vi "20- Arduino based DAQ.vi"() -> ()   [LabVIEW 2019]
uses:
  <vilib>/MakerHub/LINX/Public/Peripherals/Digital/Digital Write 1 Chan.vi
  <vilib>/MakerHub/LINX/Public/Peripherals/Analog/Analog Read 1 Chan.vi
  <vilib>/MakerHub/LINX/Public/Peripherals/Digital/Digital Write N Chans.vi
  <vilib>/MakerHub/LINX/Public/Peripherals/Analog/Analog Read N Chans.vi
  <vilib>/MakerHub/LINX/Private/Local IO/LinxDigitalWrite.vi
  <vilib>/MakerHub/LINX/Public/Utilities/Check Channel.vi
  <vilib>/MakerHub/LINX/Private/Local IO/LinxAnalogRead.vi
  <vilib>/MakerHub/LINX/Public/Utilities/Open Serial.vi
  <vilib>/MakerHub/LINX/Private/Utilties/Generate Error.vi
  <vilib>/MakerHub/LINX/LMH-LINX.lvlib
panel:
  in  "?":bool
  out "Waveform Graph":i32[](graph)
  in  "Plot data from stored value":bool
  in  "Data saving file":path
  in  "Baud Rate Override":u32
  in  "Serial Port":refnum<visa-resource-name>="N/A"
  out "Real time chart":dynamicdata(graph)
  in  "CH4":bool
  in  "CH3":bool
  in  "CH2":bool
  in  "CH1":bool
  in  "Alarm4":dbl
  in  "Alarm2":dbl
  in  "Alarm3":dbl
  in  "Alarm1":dbl
  out "Alarm4":bool
  out "Alarm3":bool
  out "Alarm2":bool
  out "Alarm1":bool
  out "CH4 value":dbl
  out "CH3 value":dbl
  out "CH2 value":dbl
  out "CH1 value":dbl
  out "CH4 meter":dbl(knob) scale=0.0..10.0
  out "CH3 meter":dbl(knob) scale=0.0..10.0
  out "CH2 meter":dbl(knob) scale=0.0..10.0
  out "CH1 meter":dbl(knob) scale=0.0..10.0
  in  "DO4":bool
  in  "DO3":bool
  in  "DO2":bool
  in  "DO1":bool
  # "ARDUINO BASED DATA ACQUISITION SYSTEM(DAQ)"
  # "Arduino configuration"
  # "Select channel"
  # "Set alarm value"
  # "Digital output"
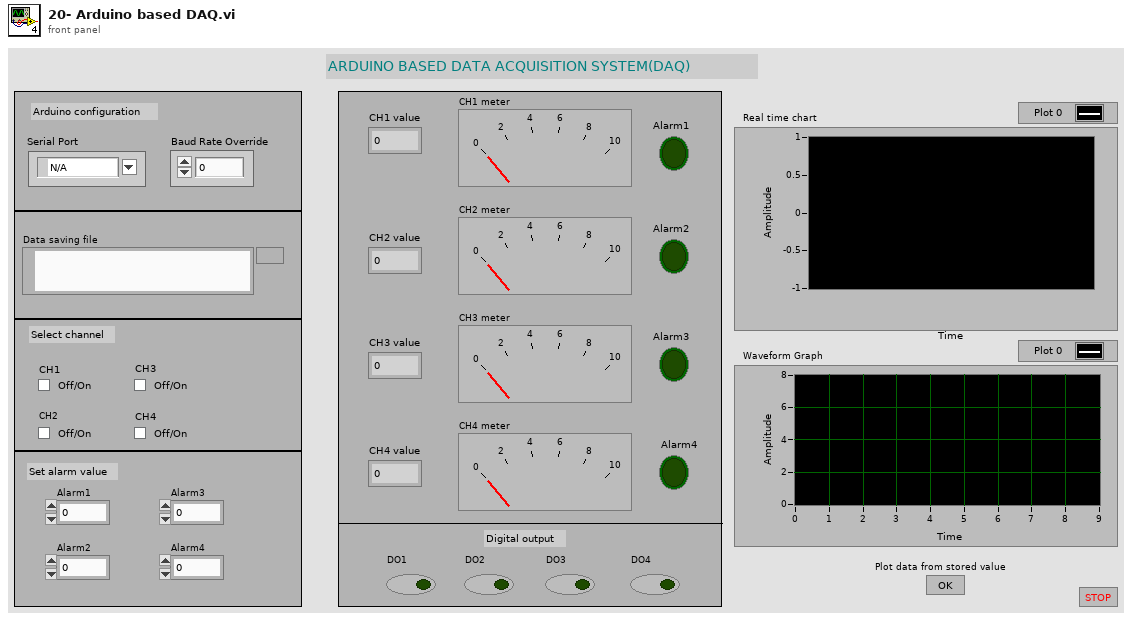
[diagram p1: front panel]
types:
  T1 = enum16{"open", "replace", "create", "open or create", "replace or create", "replace or create with confirmation"}
  T2 = typedef "LMH-LINX.lvlib/LINX Ref.ctl" = cluster{"IO":T3, "Interface":T4, "LINX Device Config":T5}
  T3 = typedef "LMH-LINX.lvlib/Platform.ctl" = enum16{"Remote", "Local"}
  T4 = typedef "LMH-LINX.lvlib/Interface.ctl" = enum16{"Serial", "TCP"}
  T5 = typedef "LMH-LINX.lvlib/Device.lvlib/LINX Device Config.ctl" = cluster{"Interface":T4, "COM Port":refnum<visa-resource-name>, "TCP Configuration":T6, "Device Family":u8, "Device ID":u8, "Device Name":string, "TCP Ref":refnum<k5>, "Channels":T7}
  T6 = typedef "LMH-LINX.lvlib/Device.lvlib/TCP Config.ctl" = cluster{"IP Address":string, "Port":u16}
  T7 = typedef "LMH-LINX.lvlib/Channels.ctl" = cluster{"DI":u8[], "DO":u8[], "AI":u8[], "AO":u8[], "PWM":u8[], "QE":u8[], "UART":u8[], "I2C 2":u8[], "SPI":u8[], "CAN":u8[], "Servo":u8[], "AI Ref (V)":dbl, "AI Resolution (Bits)":u8, "AO Ref (V)":dbl, "AO Resolution (Bits)":u8}
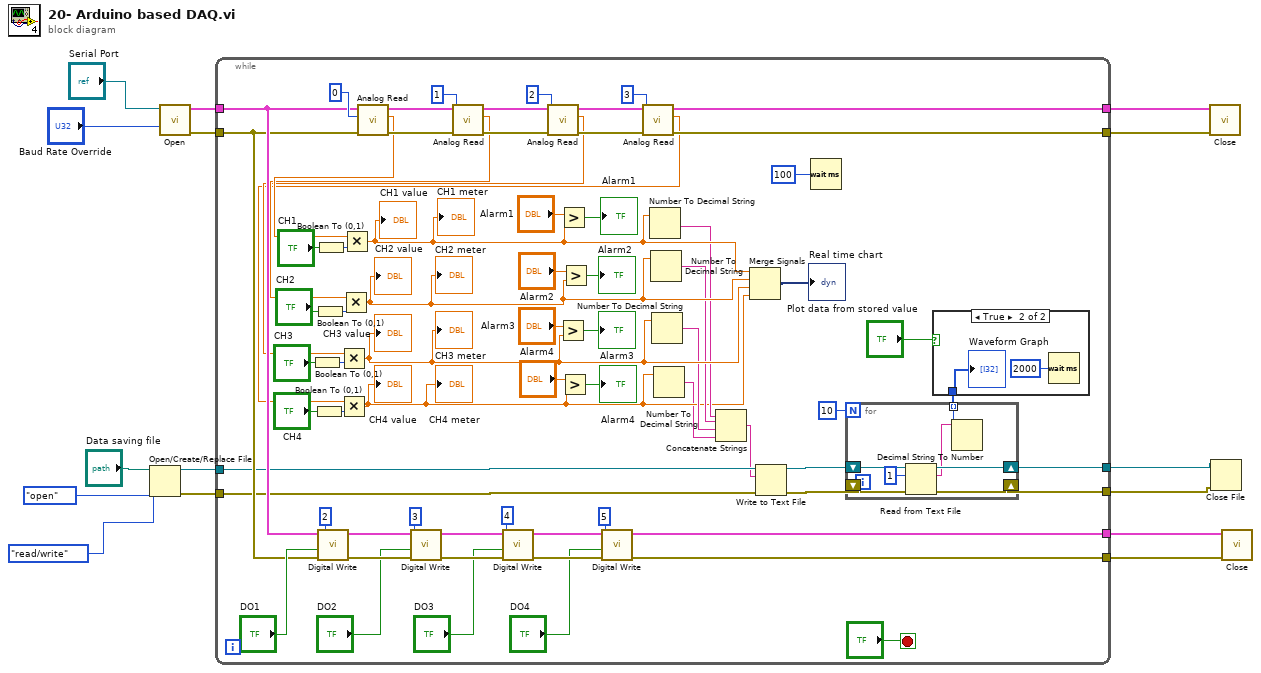
[diagram p0: block diagram]
diagram:
  n1 = Open/Create/Replace File(file path (use dialog)="Data saving file", operation (0:open)=T1."open", access (0:read/write)=enum16{"read/write", "read-only", "write-only"}."read/write") -> (refnum out=w4:refnum<file>, error out=w3:errorcluster)  [unwired: 3 in, 1 out]
  n2 = call-poly <vilib>:"Open.vi"("Baud Rate Override"="Baud Rate Override", "Serial Port"="Serial Port") -> ("Error Out"=w14:errorcluster, "LINX Resource"=w15:T2)  [unwired: 7 in, 1 out]
  n3 = while {
    tunnel: [w62] -> w9
    tunnel: w15 -> [w61]
    tunnel: w14 -> [w59]
    tunnel: [w60] -> w8
    tunnel: [w58] -> w13
    tunnel: [w57] -> w12
    tunnel: w4 -> [w35]
    tunnel: w3 -> [w34]
    tunnel: [w21] -> w2
    tunnel: [w19] -> w1
    stop <- "?" stop-if-true
    n4 = Boolean To (0,1)(Boolean="CH3") -> (0, 1=w42:i16)
    n5 = Boolean To (0,1)(Boolean="CH4") -> (0, 1=w41:i16)
    n6 = Boolean To (0,1)(Boolean="CH2") -> (0, 1=w43:i16)
    n7 = Boolean To (0,1)(Boolean="CH1") -> (0, 1=w44:i16)
    n8 = call-poly <vilib>:"Digital Write.vi"("Error In"=w59, "Output Value"="DO1", "DO Channel"=u8 2, "LINX Resource"=w61) -> ("Error Out"=w77:errorcluster, "LINX Resource"=w80:T2)  [unwired: 6 in]
    n9 = call-poly <vilib>:"Analog Read.vi"("Error In"=w59, "Analog Channel"=u8 0, "LINX Resource"=w61) -> ("Error Out"=w83:errorcluster, "Voltage"=w48:dbl, "LINX Resource"=w86:T2)  [unwired: 5 in, 1 out]
    n10 = Multiply(x=w48, y=w44) -> (x*y=w33:dbl)
    "CH1 meter" <- w33
    "CH1 value" <- w33
    n11 = call-poly <vilib>:"Digital Write.vi"("Error In"=w77, "Output Value"="DO2", "DO Channel"=u8 3, "LINX Resource"=w80) -> ("Error Out"=w76:errorcluster, "LINX Resource"=w79:T2)  [unwired: 6 in]
    n12 = call-poly <vilib>:"Analog Read.vi"("Error In"=w83, "Analog Channel"=u8 1, "LINX Resource"=w86) -> ("Error Out"=w82:errorcluster, "Voltage"=w47:dbl, "LINX Resource"=w85:T2)  [unwired: 5 in, 1 out]
    n13 = Multiply(x=w47, y=w43) -> (x*y=w32:dbl)
    "CH2 meter" <- w32
    "CH2 value" <- w32
    n14 = call-poly <vilib>:"Digital Write.vi"("Error In"=w76, "Output Value"="DO3", "DO Channel"=u8 4, "LINX Resource"=w79) -> ("Error Out"=w75:errorcluster, "LINX Resource"=w78:T2)  [unwired: 6 in]
    n15 = call-poly <vilib>:"Analog Read.vi"("Error In"=w82, "Analog Channel"=u8 2, "LINX Resource"=w85) -> ("Error Out"=w81:errorcluster, "Voltage"=w46:dbl, "LINX Resource"=w84:T2)  [unwired: 5 in, 1 out]
    n16 = Multiply(x=w46, y=w42) -> (x*y=w31:dbl)
    "CH3 meter" <- w31
    "CH3 value" <- w31
    n17 = Greater?(x="Alarm3", y=w31) -> (0:→"Alarm3":bool)
    n18 = Greater?(x="Alarm1", y=w33) -> (0:→"Alarm1":bool)
    n19 = Greater?(x="Alarm2", y=w32) -> (0:→"Alarm2":bool)
    n20 = call-poly <vilib>:"Digital Write.vi"("Error In"=w75, "Output Value"="DO4", "DO Channel"=u8 5, "LINX Resource"=w78) -> ("Error Out"=w57:errorcluster, "LINX Resource"=w58:T2)  [unwired: 6 in]
    n21 = call-poly <vilib>:"Analog Read.vi"("Error In"=w81, "Analog Channel"=u8 3, "LINX Resource"=w84) -> ("Error Out"=w60:errorcluster, "Voltage"=w45:dbl, "LINX Resource"=w62:T2)  [unwired: 5 in, 1 out]
    n22 = Multiply(x=w45, y=w41) -> (x*y=w27:dbl)
    "CH4 meter" <- w27
    "CH4 value" <- w27
    n23 = Greater?(x="Alarm4", y=w27) -> (0:→"Alarm4":bool)
    n24 = Number To Decimal String(number=w33) -> (decimal integer string=w30:string)  [unwired: 1 in]
    n25 = Number To Decimal String(number=w32) -> (decimal integer string=w29:string)  [unwired: 1 in]
    n26 = Number To Decimal String(number=w31) -> (decimal integer string=w28:string)  [unwired: 1 in]
    n27 = Number To Decimal String(number=w27) -> (decimal integer string=w26:string)  [unwired: 1 in]
    n28 = Concatenate Strings(w30, w29, w28, w26) -> (w25:string)
    n29 = Merge Signals(w33, w32, w31, w27) -> (→"Real time chart":dynamicdata)
    n30 = Write to Text File(file (use dialog)=w35, text=w25, error in=w34) -> (refnum out=w22:refnum<file>, error out=w20:errorcluster)  [unwired: 1 in, 1 out]
    n31 = Wait (ms)(milliseconds to wait=u32 100 ("millisecond timer value")) -> ()  [unwired: 1 out]
    n32 = for {
      N: 10 -> [_]
      shift-right: [w94] -> w21
      shift-left: w22 -> [w95]
      shift-right: [w92] -> w19
      shift-left: w20 -> [w93]
      tunnel: [w89] -> w16 mode=indexing
      n33 = Read from Text File(file (use dialog)=w95, count=1, error in=w93) -> (refnum out=w94:refnum<file>, text=w90:string, error out=w92:errorcluster)  [unwired: 1 in, 1 out]
      n34 = Decimal String To Number(string=w90) -> (number=w89:i32)  [unwired: 2 in, 1 out]
    }
    n35 = case shown="True" "Plot data from stored value" {
      tunnel: w16 -> [_ w88]
      frame False {
      }
      frame True {
        n36 = Wait (ms)(milliseconds to wait=u32 2000 ("millisecond timer value")) -> ()  [unwired: 1 out]
        "Waveform Graph" <- w88
      }
    }
  }
  n37 = call <vilib>:"Close.vi"("Error In"=w8, "LINX Resource"=w9) -> ()  [unwired: 9 in, 1 out]
  n38 = Close File(refnum=w2, error in=w1) -> ()  [unwired: 2 out]
  n39 = call <vilib>:"Close.vi"("Error In"=w12, "LINX Resource"=w13) -> ()  [unwired: 9 in, 1 out]
